vi "Write IsConfigured.vi"(8 "error in (no error)":errorcluster, 10 "IsConfigured?":bool, 11 "Attribute.Instrument in":refnum<class "Attribute.Instrument.lvclass">) -> (0 "error out":errorcluster, 3 "Attribute.Instrument out":refnum<class "Attribute.Instrument.lvclass">)   [LabVIEW 2019, in "Instrument Attributes.lvlib" / "Attribute.Instrument.lvclass"]
uses:
  Attribute.Instrument.lvclass
  Attribute.Instrument.lvclass/Attribute.Instrument.ctl
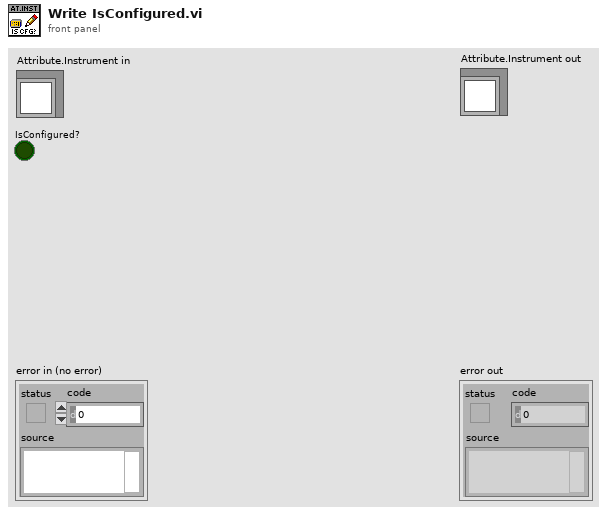
[diagram p1: front panel]
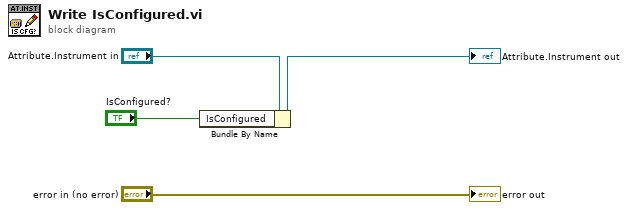
[diagram p0: block diagram]
diagram:
  n1 = Bundle By Name(cluster="Attribute.Instrument in", "IsConfigured"="IsConfigured?") -> (→"Attribute.Instrument out":refnum<class "Attribute.Instrument.lvclass">)
  "error out" <- "error in (no error)"
